vi "Read Value.vi"(8 "error in (no error)":errorcluster, 11 "Attribute in":refnum<class "Attribute.lvclass">) -> (0 "error out":errorcluster, 2 "VILab.lvlib:Data Item.lvclass":refnum<class "Data Item.lvclass">, 3 "Attribute out":refnum<class "Attribute.lvclass">)   [LabVIEW 2018, in "VILab.lvlib" / "Attribute.lvclass"]
uses:
  Attribute.lvclass
  Data Item.lvclass
  Attribute.lvclass/Attribute.ctl
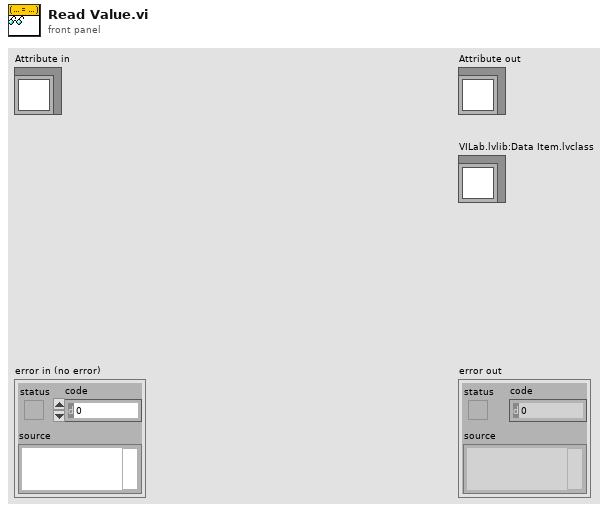
[diagram p1: front panel]
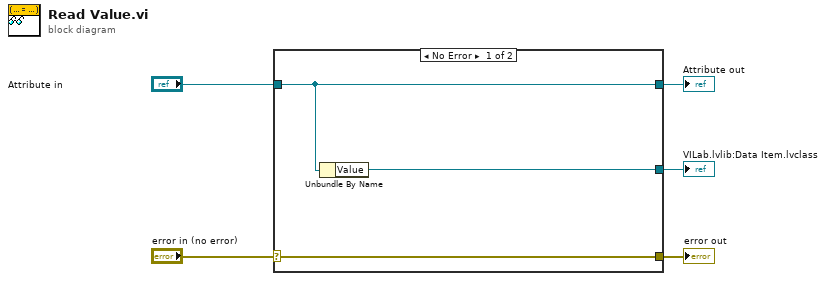
[diagram p0: block diagram]
diagram:
  n1 = case shown="No Error" "error in (no error)" {
    selector: "error in (no error)" -> [w8 w9]
    tunnel: [w8 w9] -> w4
    tunnel: [w7 w10] -> w2
    tunnel: "Attribute in" -> [w7 w10]
    tunnel: [w6 _] -> w1
    frame No Error {
      n2 = Unbundle By Name(w7) -> ("Value"=w6:refnum<class "Data Item.lvclass">)
    }
    frame Error {
    }
  }
  "error out" <- w4
  "Attribute out" <- w2
  "VILab.lvlib:Data Item.lvclass" <- w1
